vi "DSF.Engine.Framework.Get Debug Flags.vi"(11 "Framework in":refnum<class "DSF.Engine.Framework.lvclass">) -> (2 "Debug Flags":refnum<class "DSF.Engine.Debug Flags.lvclass">, 3 "Framework out":refnum<class "DSF.Engine.Framework.lvclass">)   [LabVIEW 2017, in "DSF.Engine.lvlib" / "DSF.Engine.Framework.lvclass"]
uses:
  DSF.Engine.Framework.lvclass
  Debug/DSF.Engine.Debug Flags.lvclass
  DSF.Engine.Framework.lvclass/DSF.Engine.Framework.ctl
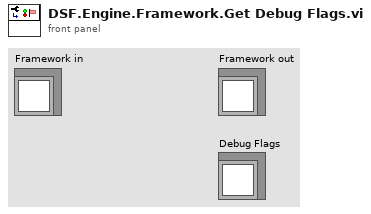
[diagram p1: front panel]
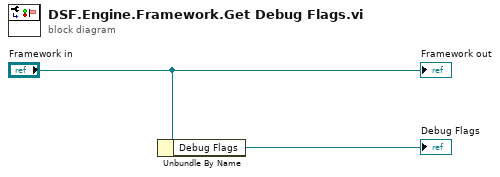
[diagram p0: block diagram]
diagram:
  n1 = Unbundle By Name("Framework in") -> ("Debug Flags"=→"Debug Flags":refnum<class "DSF.Engine.Debug Flags.lvclass">)
  "Framework out" <- "Framework in"
